vi "Modbus TCP Initialise.vi"(7 "Slave ID (255)":u8=255, 8 "error in (no error)":errorcluster, 9 "Timeout (10000)":i32=10000, 10 "Port (502)":u16=502, 11 "IP Address":string="localhost") -> (0 "error out":errorcluster, 3 "MB_TCP session":refnum<class "MB_Master_TCP.lvclass">)   [LabVIEW 2024, in "Bronkhorst Flexi-Flow ModbusTCP API.lvlib"]
uses:
  Bronkhorst Flexi-Flow ModbusTCP API.lvlib
  <vilib>/Plasmionique/MB Master/MB_Master_TCP/MB_Master_TCP.lvclass
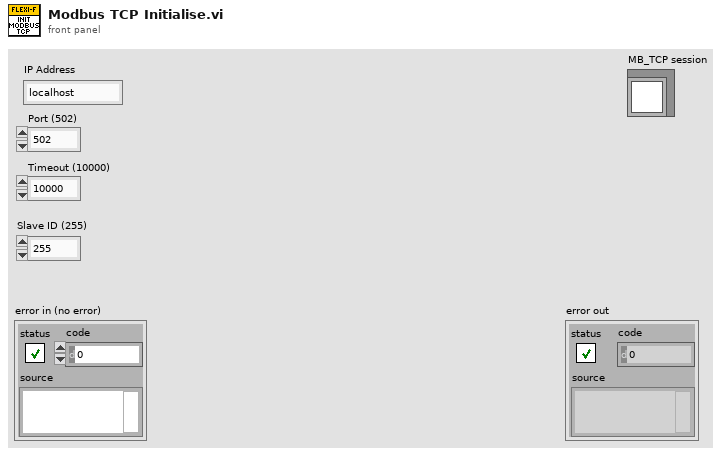
[diagram p1: front panel]
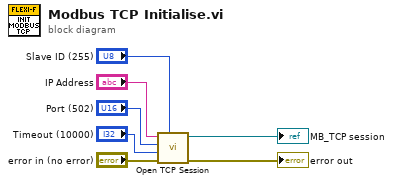
[diagram p0: block diagram]
diagram:
  n1 = call <vilib>:"Open TCP Session.vi"("Slave ID (255)"="Slave ID (255)", "error in (no error)"="error in (no error)", "Timeout (10000)"="Timeout (10000)", "Port (502)"="Port (502)", "IP Address"="IP Address") -> ("error out"=→"error out":errorcluster, "MB_TCP session"=→"MB_TCP session":refnum<class "MB_Master_TCP.lvclass">)  [unwired: 5 in]
